vi "RandomSample.vi"(6 "widthStep":dbl=500.0, 8 "error in (no error)":errorcluster, 9 "lenghtStep":dbl=500.0, 10 "basePoint":dbl[](array[numeric]), 11 "object in":refnum<class "Zone.lvclass">) -> (0 "error out":errorcluster, 2 "randomPoint":dbl[](array[numeric]), 3 "object out":refnum<class "Zone.lvclass">)   [LabVIEW 2023, in "Zone.lvclass"]
uses:
  Zone.lvclass
  <vilib>/numeric/Random Number (Range) DBL.vi
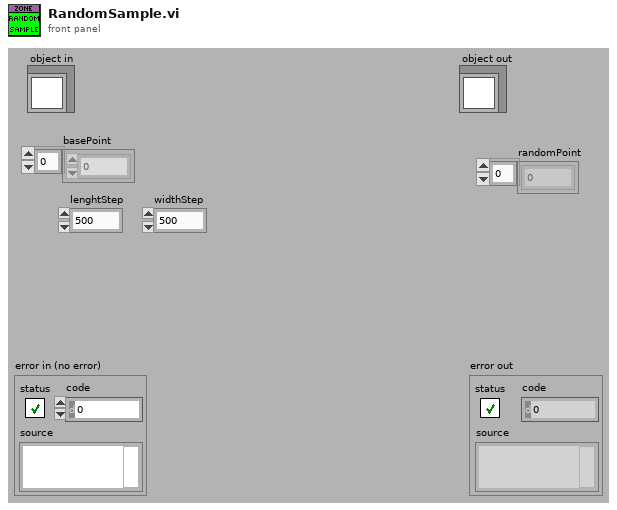
[diagram p1: front panel]
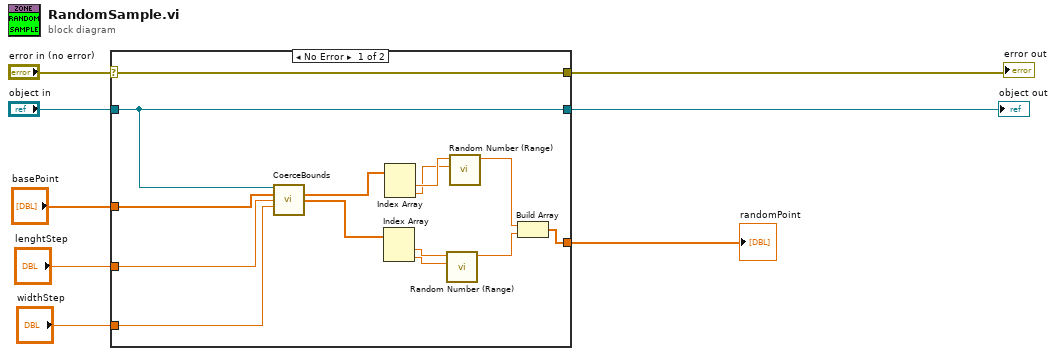
[diagram p0: block diagram]
diagram:
  n1 = case shown="No Error" "error in (no error)" {
    selector: "error in (no error)" -> [w22 w24]
    tunnel: [w22 w24] -> w7
    tunnel: [w21 w23] -> w5
    tunnel: "object in" -> [w21 w23]
    tunnel: "basePoint" -> [w20 _]
    tunnel: [w11 _] -> w3
    tunnel: "lenghtStep" -> [w10 _]
    tunnel: "widthStep" -> [w9 _]
    frame No Error {
      n2 = call-dynamic "CoerceBounds.vi"("Zone in"=w21, "centerPosition"=w20, "lenght"=w10, "width"=w9) -> ("lenghtBounds"=w19:dbl[], "widthBounds"=w16:dbl[])  [unwired: 8 in, 2 out]
      n3 = Index Array(array=w16) -> (element #1=w15:dbl, element #2=w14:dbl)  [unwired: 2 in]
      n4 = Index Array(array=w19) -> (element #1=w18:dbl, element #2=w17:dbl)  [unwired: 2 in]
      n5 = call-poly <vilib>:"Random Number (Range).vi"("lower bound (0)"=w14, "upper bound (100)"=w15) -> ("number"=w12:dbl)  [unwired: 9 in]
      n6 = call-poly <vilib>:"Random Number (Range).vi"("lower bound (0)"=w17, "upper bound (100)"=w18) -> ("number"=w13:dbl)  [unwired: 9 in]
      n7 = Build Array(w13, w12) -> (w11:dbl[])
    }
    frame Error {
    }
  }
  "error out" <- w7
  "object out" <- w5
  "randomPoint" <- w3
